vi "Abort LowMaster.vi"() -> ()   [LabVIEW 2019]
panel:
  in  "vi path":path=path "/Users/Shared/NML Data Acquisition/LowMaster/LowMaster.vi"
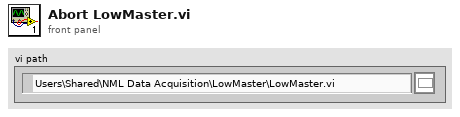
[diagram p1: front panel]
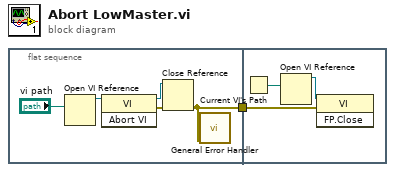
[diagram p0: block diagram]
diagram:
  n1 = flat-sequence {
    tunnel: [w2] -> w1
    tunnel: w1 -> [w7]
    frame #0 {
      n2 = Open VI Reference(vi path="vi path") -> (vi reference=w5:refnum<vi>)  [unwired: 5 in, 1 out]
      n3 = invoke class="VI" method="Abort VI"(reference=w5) -> (reference out=w4:refnum<vi>, error out=w3:errorcluster)  [unwired: 2 in, 1 out]
      n4 = Close Reference(reference=w4, error in (no error)=w3) -> (error out=w2:errorcluster)
      n5 = call <vilib>:"General Error Handler.vi"("error in (no error)"=w2) -> ()  [unwired: 10 in, 5 out]
    }
    frame #1 {
      n6 = Current VI's Path() -> (path=w9:path)
      n7 = Open VI Reference(vi path=w9) -> (vi reference=w8:refnum<vi>)  [unwired: 5 in, 1 out]
      n8 = invoke class="VI" method="FP.Close"(reference=w8, error in=w7) -> ()  [unwired: 1 in, 3 out]
    }
  }
